vi "initialize-monthly-logfile.vi"(7 "log folder":path=path "C:/Users/LocalAdmin/Documents/omicron-rack/pressure-logs", 8 "error in":errorcluster, 11 "ref in":T1 format="%.0x") -> (0 "error out":errorcluster, 3 "ref out":T1 format="%.0x")   [LabVIEW 2016]
uses:
  <vilib>/addons/h5labview2/base/hid_t.ctl
  <vilib>/addons/h5labview2/file/H5Fmode.ctl
  <vilib>/addons/h5labview2/file/H5F.lvlib
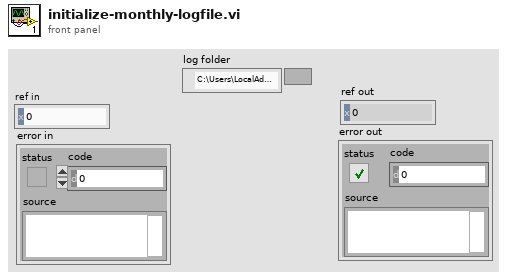
[diagram p1: front panel]
types:
  T1 = typedef "hid_t.ctl" = i32
  T2 = typedef "H5F.lvlib/H5Fmode.ctl" = enum16{"read-only", "read-write", "overwrite", "create new", "open or create"}
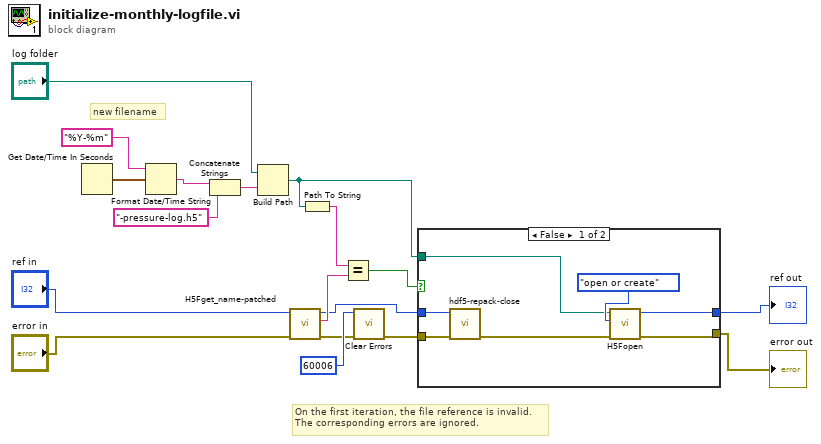
[diagram p0: block diagram]
diagram:
  # "On the first iteration, the file reference is invalid.\nThe corresponding errors are ignored."
  # "new filename"
  n1 = Get Date/Time In Seconds() -> (seconds since 1Jan1904=w18:timestamp)
  n2 = Format Date/Time String(time format string (%c)="%Y-%m", seconds (now)=w18) -> (date/time string=w16:string)  [unwired: 1 in]
  n3 = Concatenate Strings(w16, "-pressure-log.h5" ("string")) -> (w6:string)
  n4 = Build Path(base path="log folder", name or relative path=w6) -> (appended path=w5:path)
  n5 = call "H5Fget_name-patched.vi"("error in (no error)"="error in", "ref in"="ref in") -> ("error out"=w2:errorcluster, "name"=w11:string, "ref out"=w9:T1)  [unwired: 7 in]
  n6 = Path To String(path=w5) -> (string=w4:string)
  n7 = Equal?(x=w4, y=w11) -> (x = y?=w14:bool)
  n8 = call <vilib>:"Clear Errors.vi"("error in (no error)"=w2, "specific error code to clear (0: all)"=60006) -> ("error out"=w1:errorcluster)  [unwired: 4 in, 1 out]
  n9 = case shown="False" w14 {
    tunnel: [w23 w27] -> w13
    tunnel: [w24 w26] -> w12
    tunnel: w1 -> [w22 w26]
    tunnel: w9 -> [w21 w27]
    tunnel: w5 -> [w20 _]
    frame False {
      n10 = call "hdf5-repack-close.vi"("error in"=w22, "ref in"=w21) -> ("error out"=w19:errorcluster)  [unwired: 9 in]
      n11 = call <vilib>:"H5Fopen.vi"("error in (no error)"=w19, "mode (read-only)"=H5Fmode."open or create", "path"=w20) -> ("error out"=w24:errorcluster, "ref out"=w23:T1)  [unwired: 7 in]
    }
    frame True {
    }
  }
  "ref out" <- w13
  "error out" <- w12
